vi "Read Sync Mode.vi"(8 "error in (no error)":errorcluster, 11 "SPARC4_AC in":refnum<class "S4ACS_GUI.lvclass">) -> (0 "error out":errorcluster, 2 "Sync Mode":u16(ring) items=["Not Synchronized", "Continuous Mode", "Aligned by the edge", "Aligned by the center"], 3 "SPARC4_AC out":refnum<class "S4ACS_GUI.lvclass">)   [LabVIEW 2018, in "S4ACS_GUI.lvclass"]
uses:
  S4ACS_GUI.lvclass
  S4ACS_GUI.lvclass/S4ACS_GUI.ctl
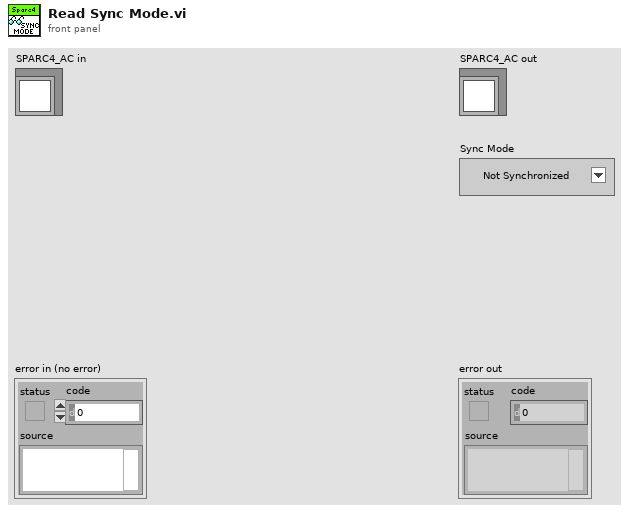
[diagram p1: front panel]
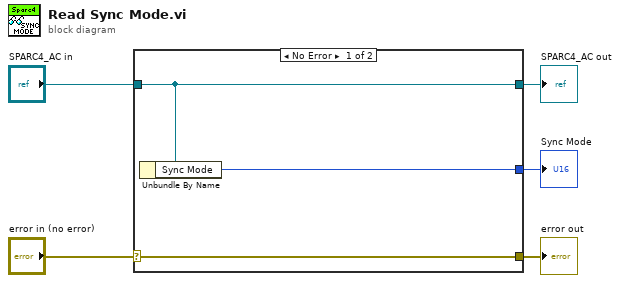
[diagram p0: block diagram]
diagram:
  n1 = case shown="No Error" "error in (no error)" {
    selector: "error in (no error)" -> [w8 w9]
    tunnel: [w8 w9] -> w4
    tunnel: [w7 w10] -> w2
    tunnel: "SPARC4_AC in" -> [w7 w10]
    tunnel: [w6 _] -> w1
    frame No Error {
      n2 = Unbundle By Name(w7) -> ("Sync Mode"=w6:u16)
    }
    frame Error {
    }
  }
  "error out" <- w4
  "SPARC4_AC out" <- w2
  "Sync Mode" <- w1
